vi "Indexing objective OG waveform.vi"(0 "Window size for layer index":dbl, 1 "OG start layer":dbl, 2 "OG end layer":dbl, 3 "Steps per Volume":dbl, 4 "OG repitation":dbl, 5 "Waveform":waveform(dbl), 7 "OG Z 线性加速 采样信息":cluster{"采样率":dbl, "采样数":dbl}, 9 "OG Z stack 刺激 steps 采样信息":cluster{"采样率":dbl, "采样数":dbl}, 11 "OG Z volet 线性减速 采样信息":cluster{"采样率":dbl, "采样数":dbl}, 13 "OG Z 线性减速 采样信息":cluster{"采样率":dbl, "采样数":dbl}) -> (14 "Waveform_Digital":digitalwaveform(waveform)={"t0"=timestamp(0 s since 1904-01-01), "dt"=0.0, "Y"={"transitions"=[], "data"=[]}, "error"={"status"=FALSE, "code"=37421928, "source"=""}})   [LabVIEW 2018]
uses:
  <vilib>/Waveform/DWDTOps.llb/DWDT Analog to Digital.vi
  <vilib>/measure/NI_MABase.lvlib
panel:
  out "Wrong step number detected!":bool
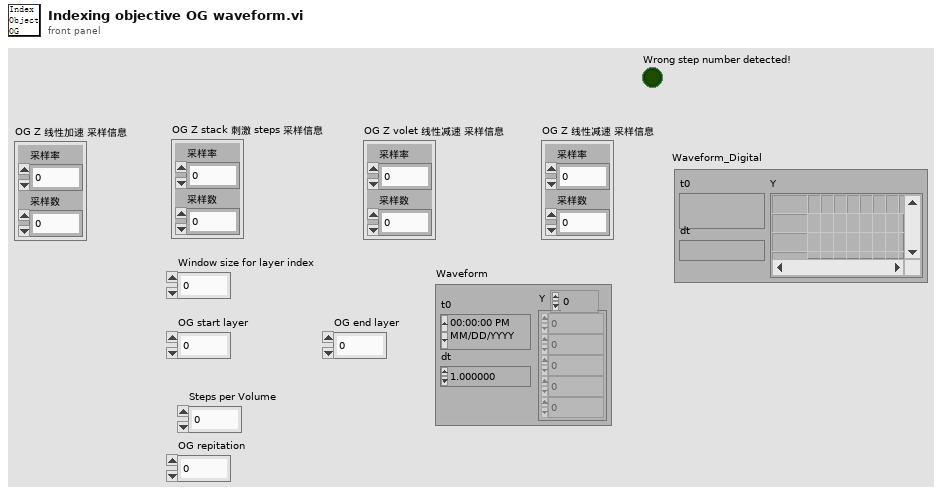
[diagram p1: front panel]
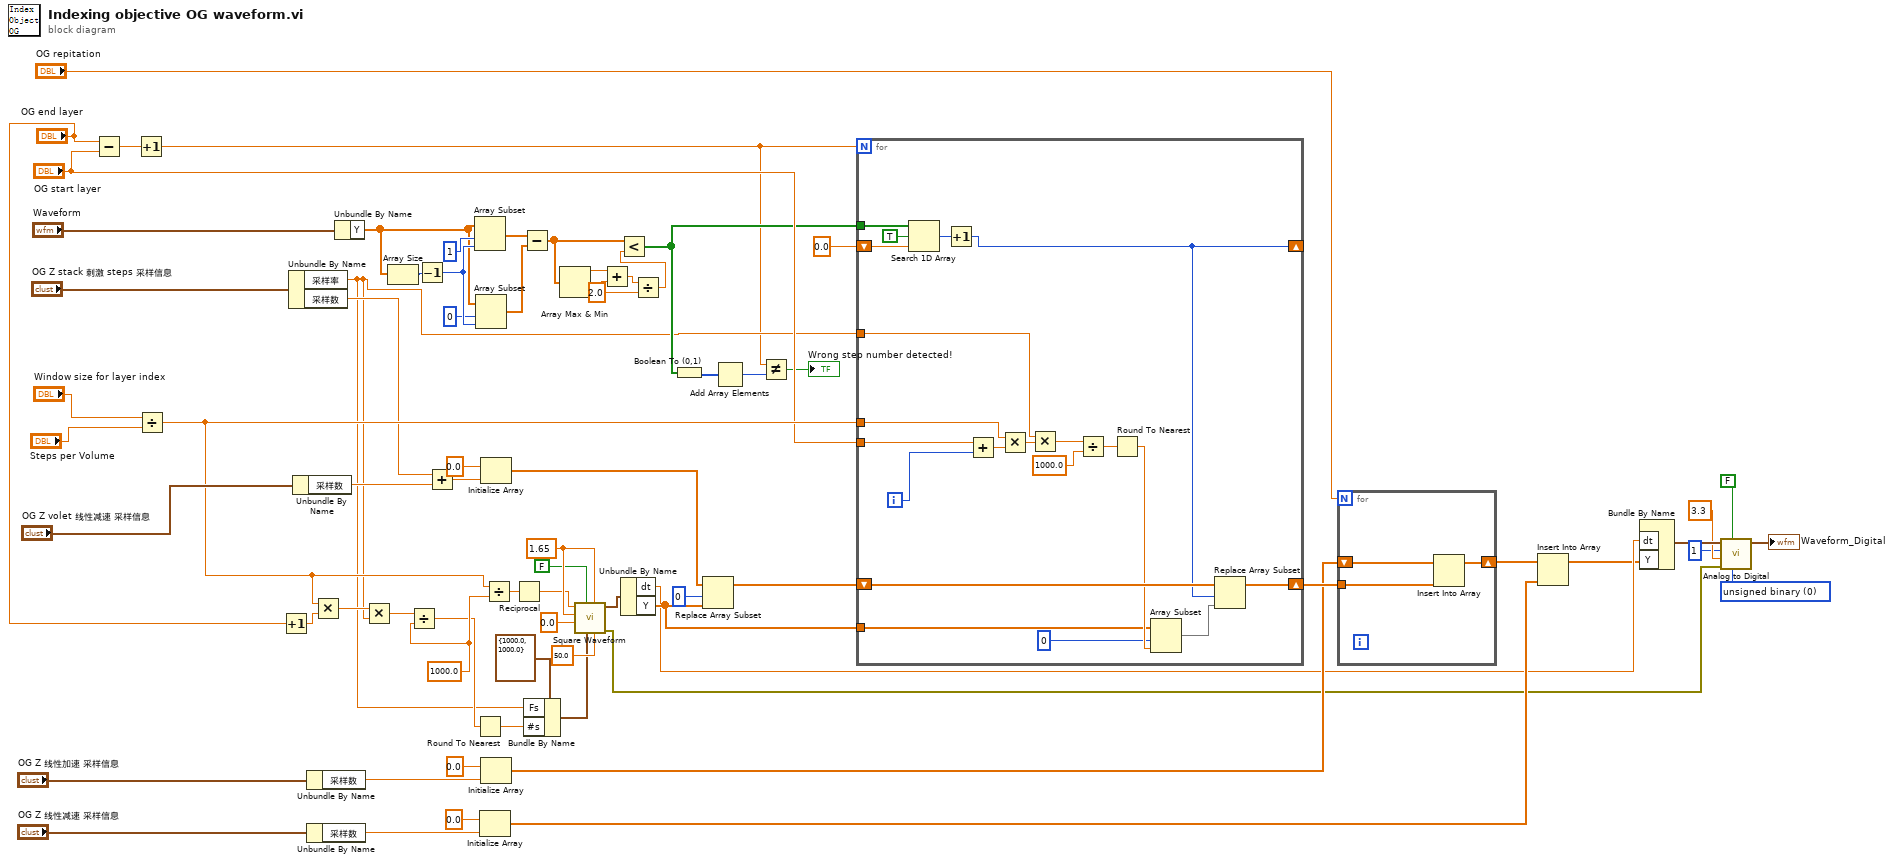
[diagram p0: block diagram]
diagram:
  w7 = u16 0 items=["unsigned binary", "offset binary", "2's complement"] ("data format (offset binary)")
  w56 = 1.65
  w50 = 1000.0 ("y")
  n1 = Subtract(x="OG end layer", y="OG start layer") -> (x-y=w69:dbl)
  n2 = Increment(x=w69) -> (x+1=w28:dbl)
  n3 = Divide(x="Window size for layer index", y="Steps per Volume") -> (x/y=w67:dbl)
  n4 = Increment(x="OG end layer") -> (x+1=w53:dbl)
  n5 = Unbundle By Name("OG Z stack 刺激 steps 采样信息") -> ("采样率"=w32:dbl, "采样数"=w62:dbl)
  n6 = Unbundle By Name("OG Z volet 线性减速 采样信息") -> ("采样数"=w63:dbl)
  n7 = Unbundle By Name("OG Z 线性加速 采样信息") -> ("采样数"=w25:dbl)
  n8 = Unbundle By Name("OG Z 线性减速 采样信息") -> ("采样数"=w24:dbl)
  n9 = Multiply(x=w67, y=w53) -> (x*y=w52:dbl)
  n10 = Unbundle By Name("Waveform") -> ("Y"=w39:dbl[])
  n11 = Multiply(x=w52, y=w32) -> (x*y=w51:dbl)
  n12 = Array Size(array=w39) -> (size(s)=w42:i32)
  n13 = Divide(x=w51, y=w50) -> (x/y=w48:dbl)
  n14 = Decrement(x=w42) -> (x-1=w43:i32)
  n15 = Add(x=w62, y=w63) -> (x+y=w61:dbl)
  n16 = Array Subset(array=w39, index=1, length=w43) -> (w37:dbl[])
  n17 = Round To Nearest(number=w48) -> (nearest integer value=w49:dbl)
  n18 = Array Subset(array=w39, index=0, length=w43) -> (w38:dbl[])
  n19 = Initialize Array(0.0 ("element"), w24) -> (w19:dbl[])
  n20 = Initialize Array(0.0 ("element"), w61) -> (w45:dbl[])
  n21 = Initialize Array(0.0 ("element"), w25) -> (w21:dbl[])
  n22 = Divide(x=w67, y=w50) -> (x/y=w57:dbl)
  n23 = Reciprocal(x=w57) -> (1/x=w8:dbl)
  n24 = Subtract(x=w37, y=w38) -> (x-y=w12:dbl[])
  n25 = Bundle By Name(cluster=cluster{"Fs":dbl, "#s":dbl} {"Fs"=1000.0, "#s"=1000.0} ("sampling info"), "Fs"=w32, "#s"=w49) -> (w47:cluster{"Fs":dbl, "#s":dbl})
  n26 = Array Max & Min(array=w12) -> (max value=w14:dbl, min value=w13:dbl)  [unwired: 2 out]
  n27 = call <vilib>:"Square Waveform.vi"("duty cycle (%)"=50.0, "offset"=w56, "sampling info"=w47, "reset signal"=FALSE, "phase"=0.0, "amplitude"=w56, "frequency"=w8) -> ("error out"=w17:errorcluster, "signal out"=w46:waveform(dbl))  [unwired: 3 in]
  n28 = Add(x=w14, y=w13) -> (x+y=w11:dbl)
  n29 = Unbundle By Name(w46) -> ("dt"=w18:dbl, "Y"=w31:dbl[])
  n30 = Divide(x=w11, y=2.0) -> (x/y=w9:dbl)
  n31 = Less?(x=w12, y=w9) -> (x < y?=w35:bool[])
  n32 = Boolean To (0,1)(Boolean=w35) -> (0, 1=w34:i16[])
  n33 = Replace Array Subset(array=w45, new element=w31, index=0) -> (w33:dbl[])
  n34 = Add Array Elements(numeric array=w34) -> (sum=w29:i16)
  n35 = Not Equal?(x=w28, y=w29) -> (x != y?=→"Wrong step number detected!":bool)
  n36 = for {
    N: w28 -> [_]
    tunnel: w67 -> [w81]
    tunnel: "OG start layer" -> [w80]
    tunnel: w35 -> [w91]
    shift-right: [w76] -> w30
    shift-left: w33 -> [w84]
    tunnel: w32 -> [w82]
    tunnel: w31 -> [w78]
    shift-right: [w74] -> _
    shift-left: 0.0 -> [w90]
    i -> [w83]
    n37 = Search 1D Array(1D array=w91, element=TRUE, start index (0)=w90) -> (index of element=w75:i32)
    n38 = Increment(x=w75) -> (x+1=w74:i32)
    n39 = Add(x=w80, y=w83) -> (x+y=w88:dbl)
    n40 = Multiply(x=w81, y=w88) -> (x*y=w89:dbl)
    n41 = Multiply(x=w82, y=w89) -> (x*y=w86:dbl)
    n42 = Divide(x=w86, y=1000.0) -> (x/y=w87:dbl)
    n43 = Round To Nearest(number=w87) -> (nearest integer value=w79:dbl)
    n44 = Array Subset(array=w78, index=0, length=w79) -> (w73:dbl[])
    n45 = Replace Array Subset(array=w84, new element=w73, index=w74) -> (w76:dbl[])
  }
  n46 = for {
    N: "OG repitation" -> [_]
    tunnel: w30 -> [w95]
    shift-right: [w93] -> w20
    shift-left: w21 -> [w94]
    n47 = Insert Into Array(array=w94, new element=w95) -> (w93:dbl[])  [unwired: 1 in]
  }
  n48 = Insert Into Array(array=w20, new element=w19) -> (w5:dbl[])  [unwired: 1 in]
  n49 = Bundle By Name("dt"=w18, "Y"=w5) -> (w4:waveform(dbl))  [unwired: 1 in]
  n50 = call-poly <vilib>:"Analog to Digital.vi"("data format (offset binary)"=w7, "compress digital (T)"=FALSE, "error in (no error)"=w17, "full-scale range (pk-pk)"=3.3, "resolution (16 bit)"=1, "analog waveform"=w4) -> ("digital waveform"=→"Waveform_Digital":digitalwaveform)  [unwired: 2 in, 3 out]
